vi "_Veritech_LVCM_Item_OnUnselect.vi"(11 "Object":T1) -> ()   [LabVIEW 2014]
uses:
  <resource>/Framework/Providers/API/ItemRef.ctl
  Support/Framework/ItemSelection/ItemSelection.lvlib
panel:
  out "error out":errorcluster
  in  "error in":errorcluster
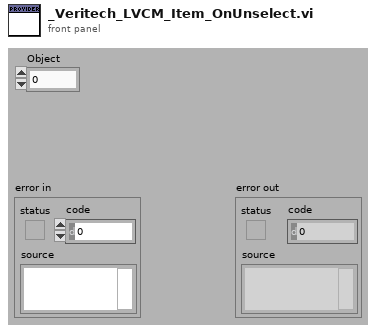
[diagram p1: front panel]
types:
  T1 = typedef "ItemRef.ctl" = u64
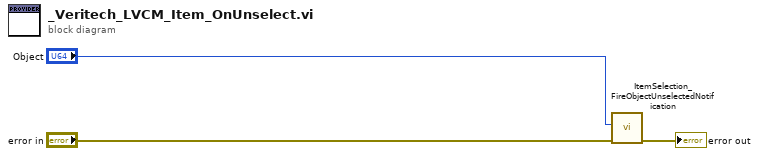
[diagram p0: block diagram]
diagram:
  n1 = call "ItemSelection_FireObjectUnselectedNotification.vi"("error in (no error)"="error in", "Object"="Object") -> ("error out"=→"error out":errorcluster)  [unwired: 9 in]
